vi "Prompt to Confirm Archival.vi"(10 "files to be deleted":path[](array[path]), 11 "archive destination":path) -> (3 "confirmed?":bool)   [LabVIEW 2020]
panel:
  in  "prompt message":string="The following files/folders must be removed to use this project. The existing files will be archived to %s.\n\n%s"
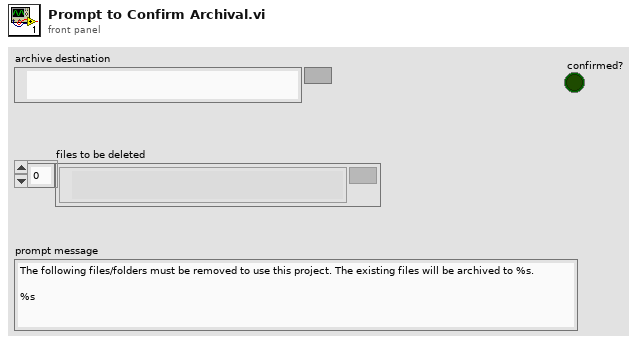
[diagram p1: front panel]
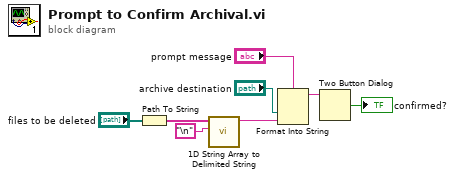
[diagram p0: block diagram]
diagram:
  n1 = Path To String(path="files to be deleted") -> (string=w2:string[])
  n2 = call <vilib>:"1D String Array to Delimited String.vi"("delimiter"="\n", "string array"=w2) -> ("delimited string"=w4:string)  [unwired: 9 in]
  n3 = Format Into String(format string="prompt message", "archive destination", w4) -> (resulting string=w5:string)  [unwired: 2 in, 1 out]
  n4 = Two Button Dialog(message=w5) -> (T button?=→"confirmed?":bool)  [unwired: 2 in]
